vi "Main.vi"() -> ()   [LabVIEW 2020]
uses:
  OXYGEN/VIs/Setup/TypeDefs/States.ctl
  OXYGEN/VIs/Channel List Access/SubVIs/ChannelList_GetNames.vi
  OXYGEN/VIs/Data Aquasation/SubVIs/GetDataPackage_Double.vi
  OXYGEN_Datastream.lvlib
panel:
  out "State":T1
  out "Channel List":cluster{"ID":string, "Name":string}[](array[cluster])
  out "XY Graph 2":T2(graph)
  in  "Configure Channels":string[](array[string])=["AI 1/I1 Sim", "AI 1/I2 Sim", "AI 1/I3 Sim", "AI 1/I4 Sim"]
  in  "stop":bool
  out "error out":errorcluster
  out "Iteration":i32
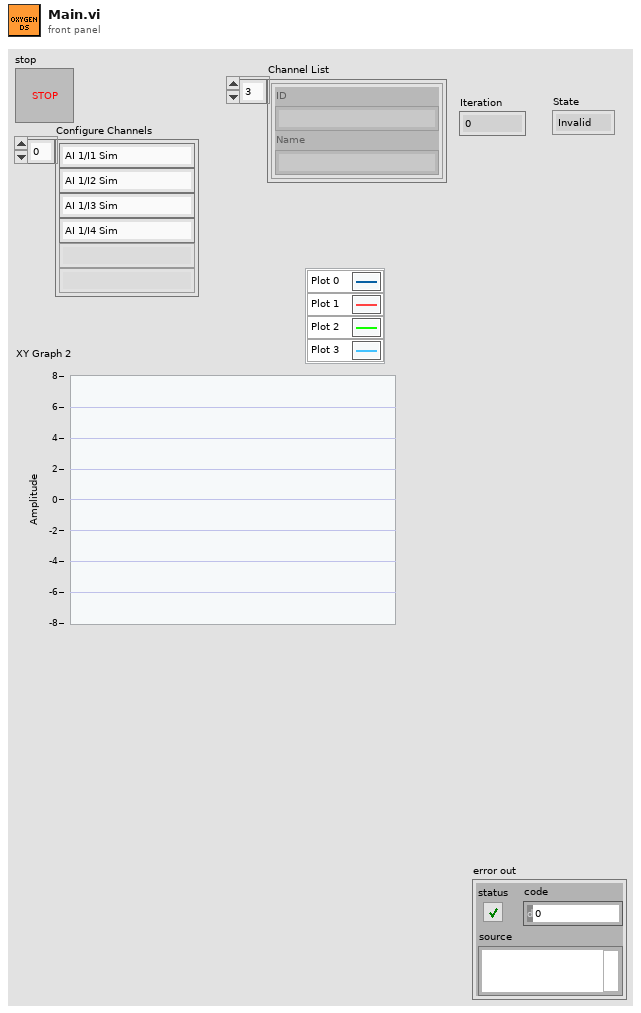
[diagram p1: front panel]
types:
  T1 = typedef "OXYGEN_Datastream.lvlib/States.ctl" = enum16{"Invalid", "Config", "Initialized", "Running", "Error", "Unlicensed"}
  T2 = cluster{"data_point":cluster{"X":dbl, "Y":dbl}[]}[]
  T3 = typedef "OXYGEN_Datastream.lvlib/DataPoint_Double.ctl" = cluster{"DataPoints":cluster{"Time":dbl, "Value":dbl}[]}
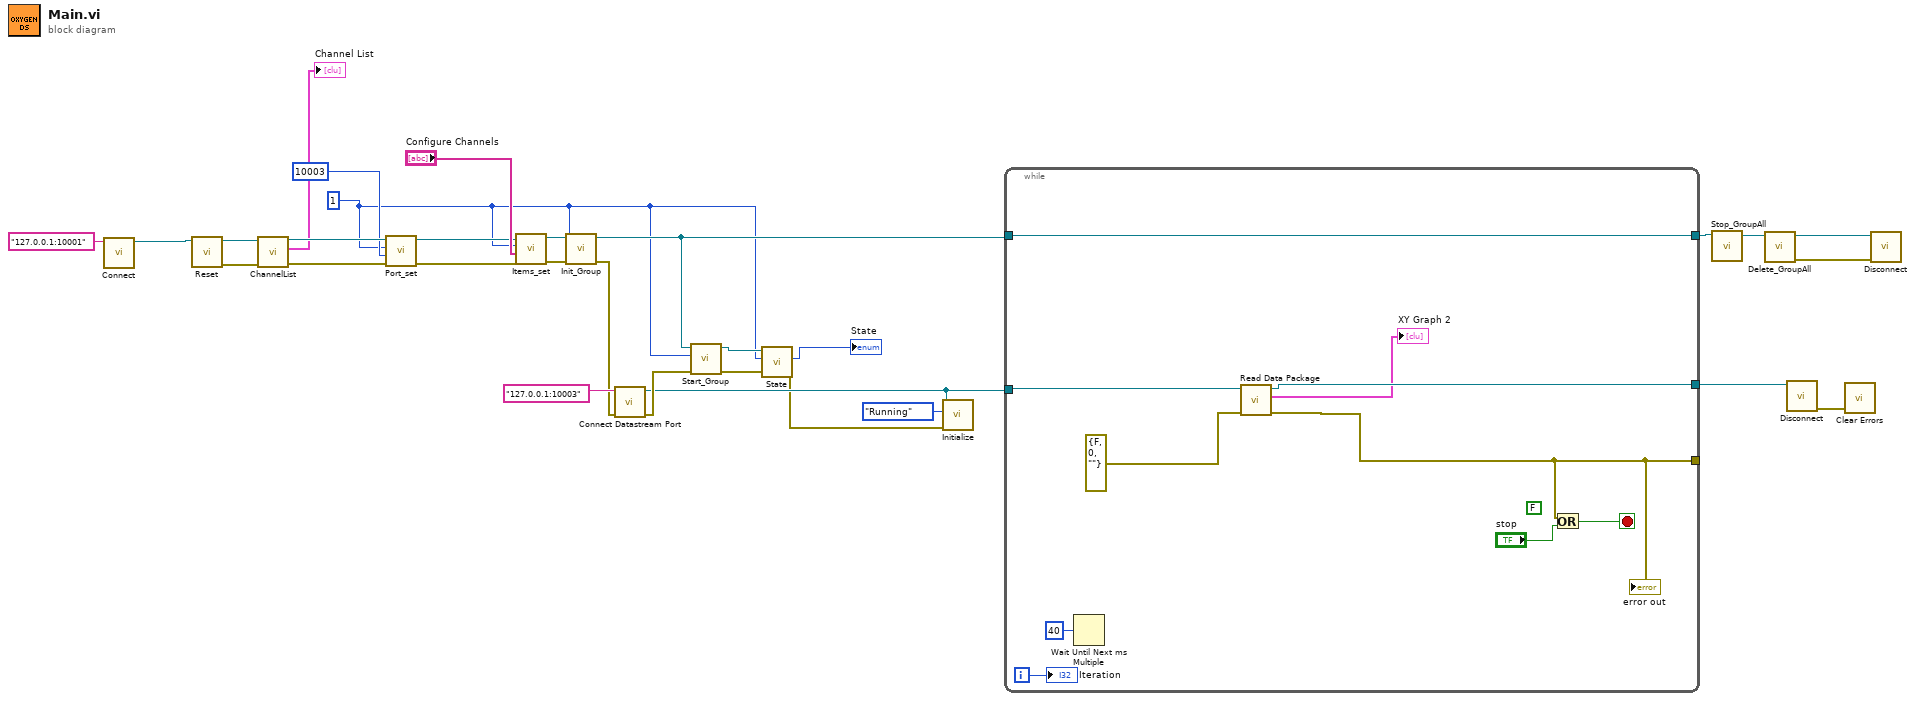
[diagram p0: block diagram]
diagram:
  w3 = 1 ("Stream Group")
  n1 = call "Connect.vi"("OXY_SCPI Resource In"="127.0.0.1:10001" ("OXY_SCPI TCP-IP address")) -> ("OXY_SCPI Resource Out"=w28:refnum<visa-resource-name>)  [unwired: 9 in, 1 out]
  n2 = call "Reset.vi"("OXY_SCPI Reseource In"=w28) -> ("error out"=w26:errorcluster, "OXY_SCPI Reseource Out"=w27:refnum<visa-resource-name>)  [unwired: 8 in, 1 out]
  n3 = call-poly "ChannelList.vi"("error in (no error)"=w26, "OXY_SCPI Reseource In"=w27) -> ("error out"=w21:errorcluster, "Channels"=→"Channel List":cluster{"ID":string, "Name":string}[], "OXY_SCPI Reseource Out"=w25:refnum<visa-resource-name>)  [unwired: 6 in, 1 out]
  n4 = call "Port_set.vi"("error in (no error)"=w21, "Port"=10003, "Stream Group"=w3, "OXY_SCPI Reseource In"=w25) -> ("error out"=w22:errorcluster, "OXY_SCPI Reseource Out"=w24:refnum<visa-resource-name>)  [unwired: 5 in, 1 out]
  n5 = call "Items_set.vi"("error in (no error)"=w22, "Channels"="Configure Channels", "Stream Group"=w3, "OXY_SCPI Reseource In"=w24) -> ("error out"=w19:errorcluster, "OXY_SCPI Reseource Out"=w20:refnum<visa-resource-name>)  [unwired: 5 in, 1 out]
  n6 = call "Init_Group.vi"("error in (no error)"=w19, "Stream Group"=w3, "OXY_SCPI Reseource In"=w20) -> ("error out"=w1:errorcluster, "OXY_SCPI Reseource Out"=w8:refnum<visa-resource-name>)  [unwired: 6 in, 1 out]
  n7 = call "Connect Datastream Port.vi"("error in (no error)"=w1, "OXY_SCPI Resource In"="127.0.0.1:10003" ("OXY_SCPI TCP-IP address")) -> ("error out"=w10:errorcluster, "OXY_SCPI Resource Out"=w9:refnum<visa-resource-name>)  [unwired: 8 in]
  n8 = call "Start_Group.vi"("error in (no error)"=w10, "Stream Group"=w3, "OXY_SCPI Reseource In"=w8) -> ("error out"=w6:errorcluster, "OXY_SCPI Reseource Out"=w7:refnum<visa-resource-name>)  [unwired: 6 in, 1 out]
  n9 = call "State.vi"("error in (no error)"=w6, "Group"=w3, "OXY_SCPI Reseource In"=w7) -> ("error out"=w5:errorcluster, "State"=→"State":T1)  [unwired: 5 in, 2 out]
  n10 = call "Initialize.vi"("error in (no error)"=w5, "Datastrem State"=States."Running", "OXY_SCPI Resource In"=w9) -> ()  [unwired: 7 in, 2 out]
  n11 = while {
    tunnel: w9 -> [w33]
    tunnel: [w34] -> _
    tunnel: w8 -> [w36]
    tunnel: [w36] -> w18
    tunnel: [w32] -> w11
    i -> [w39]
    stop <- w38 stop-if-true
    (unwired) FALSE ("x")
    n12 = Wait Until Next ms Multiple(millisecond multiple=u32 40) -> ()  [unwired: 1 out]
    n13 = call-poly "Read Data Package.vi"("error in (no error)"=errorcluster {"status"=FALSE, "code"=0, "source"=""}, "VISA Refnum in"=w33) -> ("error out"=w34:errorcluster, "Data"=→"XY Graph 2":T3[], "VISA Refnum out"=w32:refnum<visa-resource-name>)  [unwired: 6 in, 1 out]
    "error out" <- w34
    n14 = Or(x=w34, y="stop") -> (x .or. y?=w38:bool)
    "Iteration" <- w39
  }
  n15 = call "Stop_GroupAll.vi"("OXY_SCPI Reseource In"=w18) -> ("OXY_SCPI Reseource Out"=w17:refnum<visa-resource-name>)  [unwired: 8 in, 2 out]
  n16 = call "Delete_GroupAll.vi"("OXY_SCPI Reseource In"=w17) -> ("error out"=w15:errorcluster, "OXY_SCPI Reseource Out"=w16:refnum<visa-resource-name>)  [unwired: 8 in, 1 out]
  n17 = call "Disconnect.vi"("OXY_SCPI Reseource Out"=w11) -> ("error out"=w14:errorcluster)  [unwired: 10 in]
  n18 = call <vilib>:"Clear Errors.vi"("error in (no error)"=w14) -> ()  [unwired: 5 in, 2 out]
  n19 = call "Disconnect.vi"("error in (no error)"=w15, "OXY_SCPI Reseource Out"=w16) -> ()  [unwired: 9 in, 1 out]
